vi "E710_ErrorCheck.vi"(0 "Position":dbl[](array[numeric]) format="%.6f", 1 "Conn. Axes":string[](array[string]), 2 "ATZ successful?":bool[](array[boolean]), 3 "Identification":string, 7 "error out 2":errorcluster) -> (13 "error out":errorcluster)   [LabVIEW 2011]
uses:
  Variables/GlobalGetPhysikalInstrumentsOnOff.vi
  Variables/ScannerMirrorStatus.vi
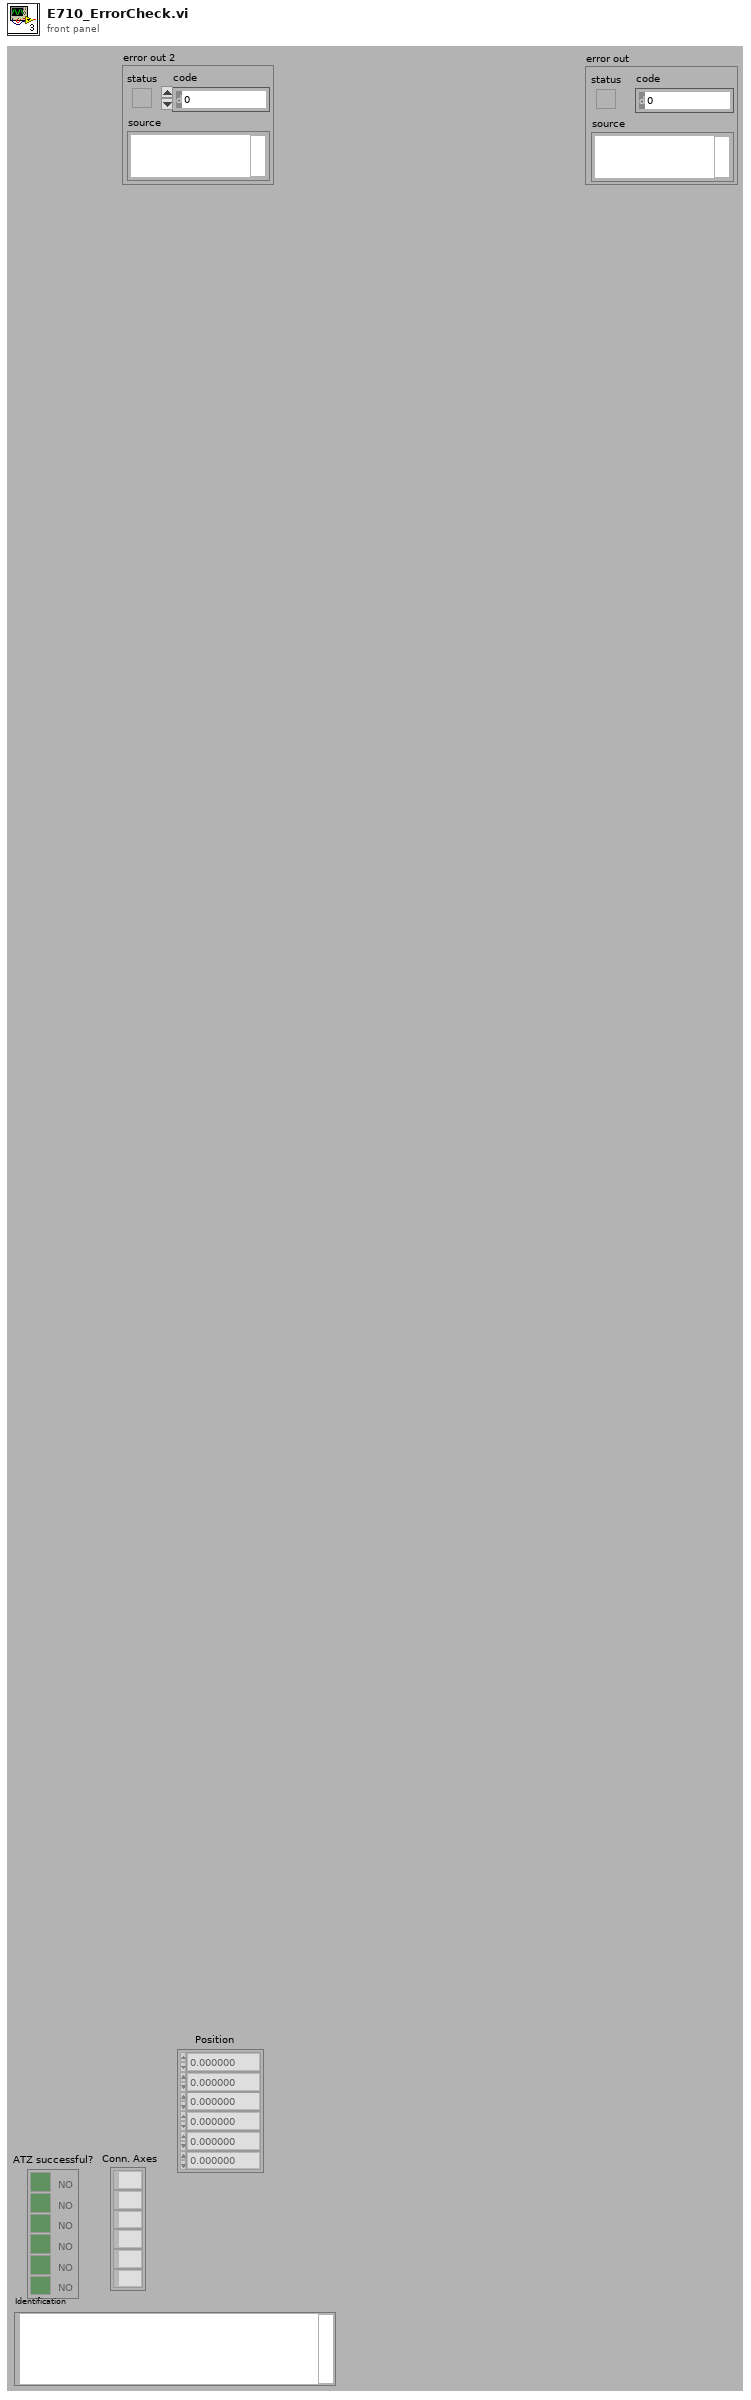
[diagram p1: front panel]
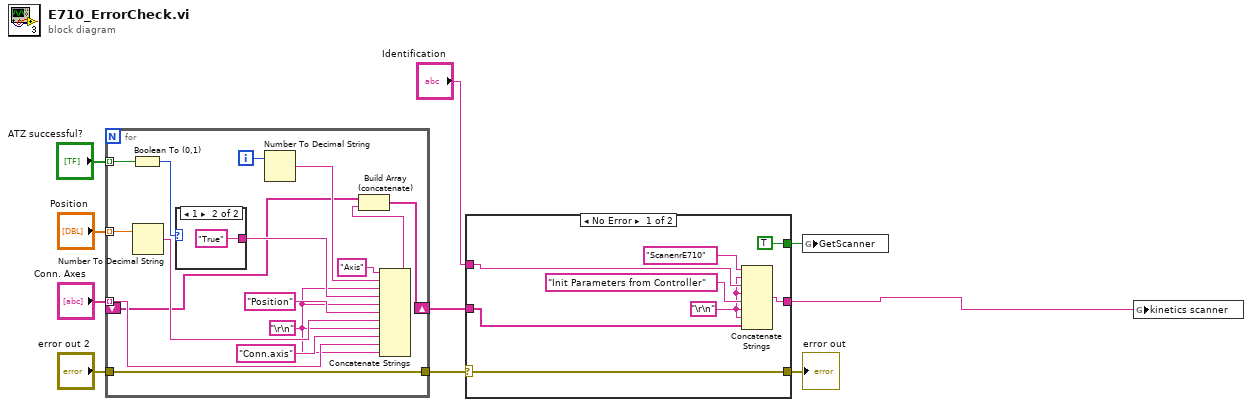
[diagram p0: block diagram]
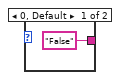
[diagram p2: hidden frame]
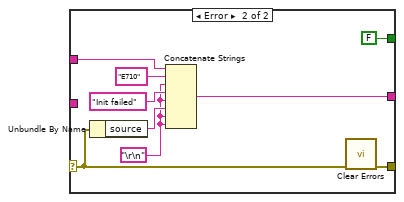
[diagram p3: hidden frame]
diagram:
  n1 = for {
    tunnel: "ATZ successful?" -> [w23] mode=indexing
    tunnel: "error out 2" -> [w20]
    tunnel: [w20] -> w4
    tunnel: "Position" -> [w18] mode=indexing
    tunnel: "Conn. Axes" -> [w15] mode=indexing
    shift-right: [w13] -> w6
    shift-left: _ -> [w11]
    i -> [w26]
    w14 = "\r\n"
    n2 = Boolean To (0,1)(Boolean=w23) -> (0, 1=w22:i16)
    n3 = Number To Decimal String(number=w18) -> (decimal integer string=w17:string)  [unwired: 1 in]
    n4 = case shown="1" w22 {
      tunnel: ["False" "True"] -> w21
      frame 0, Default {
      }
      frame 1 {
      }
    }
    n5 = Number To Decimal String(number=w26) -> (decimal integer string=w25:string)  [unwired: 1 in]
    n6 = Concatenate Strings("Axis", w25, w14, w21, w14, "Position" ("string"), w17, w14, "Conn.axis" ("string"), w15, w14) -> (w12:string)
    n7 = Build Array (concatenate)(w11, w12) -> (w13:string[])
  }
  n8 = case shown="No Error" w4 {
    selector: w4 -> [w34 w40]
    tunnel: [w35 w42] -> w1
    tunnel: [w34 w41] -> w10
    tunnel: [TRUE ("Value") FALSE ("Value")] -> w9
    tunnel: "Identification" -> [w32 w37]
    tunnel: w6 -> [w30 _]
    frame No Error {
      w29 = "\r\n"
      n9 = Concatenate Strings("ScanenrE710" ("Terminal Init 2"), w29, w32, w29, "Init Parameters from Controller" ("string"), w29, w29, w30) -> (w35:string)
    }
    frame Error {
      w39 = "\r\n"
      n10 = Unbundle By Name(w40) -> ("source"=w44:string)
      n11 = Concatenate Strings(w37, "E710" ("string"), w39, "Init failed" ("string"), w39, w44, w39, w39) -> (w42:string)
      n12 = call <vilib>:"Clear Errors.vi"("error in (no error)"=w40) -> ("error out"=w41:errorcluster)  [unwired: 6 in]
    }
  }
  "error out" <- w10
  n13 = global write "GlobalGetPhysikalInstrumentsOnOff.vi" "GetScanner"(w9) -> ()
  n14 = global write "ScannerMirrorStatus.vi" "kinetics scanner"(w1) -> ()
